vi "GamePanel.vi"() -> ()   [LabVIEW 2025]
uses:
  common/types/network/Move.ctl
  <vilib>/Utility/miscctls.llb/LVPointTypeDef.ctl
  common/types/network/FieldData.ctl
  common/types/network/FoggedFieldCell.ctl
  server/types/TerrainEnum.ctl
  common/types/network/ClientSendData.ctl
  b634419e-299d-4ea9-b051-81e51aeb9912.vi
  d835d933-86fe-443f-b748-a417a8161ed5.vi
  ClientGlobalVariables.vi
panel:
  out "Chain Move":bool=TRUE
  out "MoveSet":set{T1}(c389)
  out "Split":bool=TRUE
  out "CurrentSelectedCell":cluster{"row":i32, "col":i32}
  out "Round Number":dbl
  out "Field Display":picture
  # "Round #"
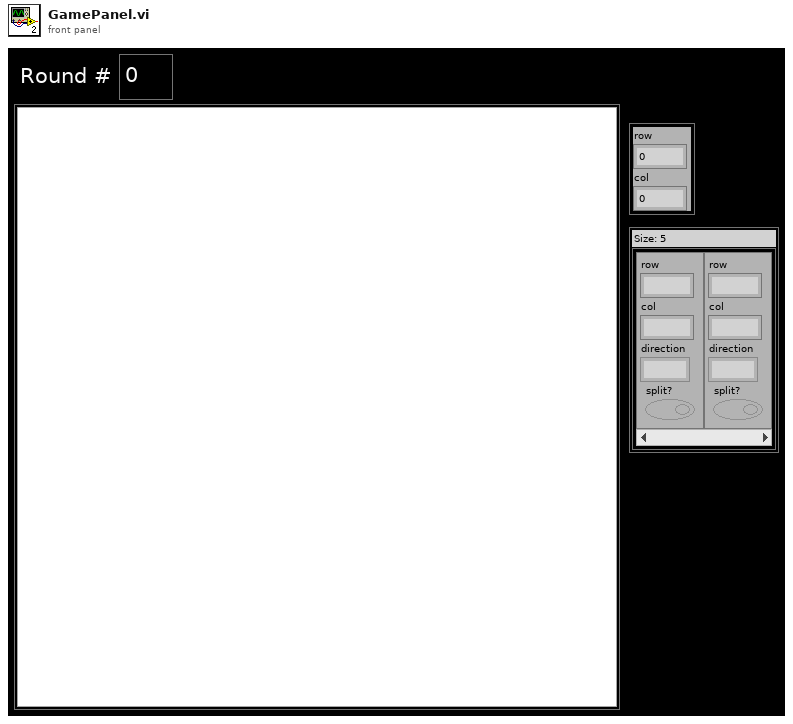
[diagram p1: front panel]
types:
  T1 = typedef "Move.ctl" = cluster{"row":u32, "col":u32, "direction":enum16{"right", "down", "left", "up"}, "split?":bool}
  T2 = typedef "LVPointTypeDef.ctl" = cluster{"Horizontal":i16, "Vertical":i16}
  T3 = typedef "LVPoint32TypeDef.ctl" = cluster{"Horizontal":i32, "Vertical":i32}
  T4 = typedef "LVPositionTypeDef.ctl" = cluster{"Left":i32, "Top":i32}
  T5 = typedef "TerrainEnum.ctl" = enum16{"Plain", "Mountain", "City", "General"}
  T6 = typedef "FoggedFieldCell.ctl" = cluster{"Troops":u32, "Owner":i32, "Terrain":T5, "Fog":bool}
  T7 = typedef "FieldData.ctl" = cluster{"Round":u32, "FoggedFieldArray":T6[][]}
  T8 = typedef "ClientSendData.ctl" = cluster{"Action":string, "Data":string}
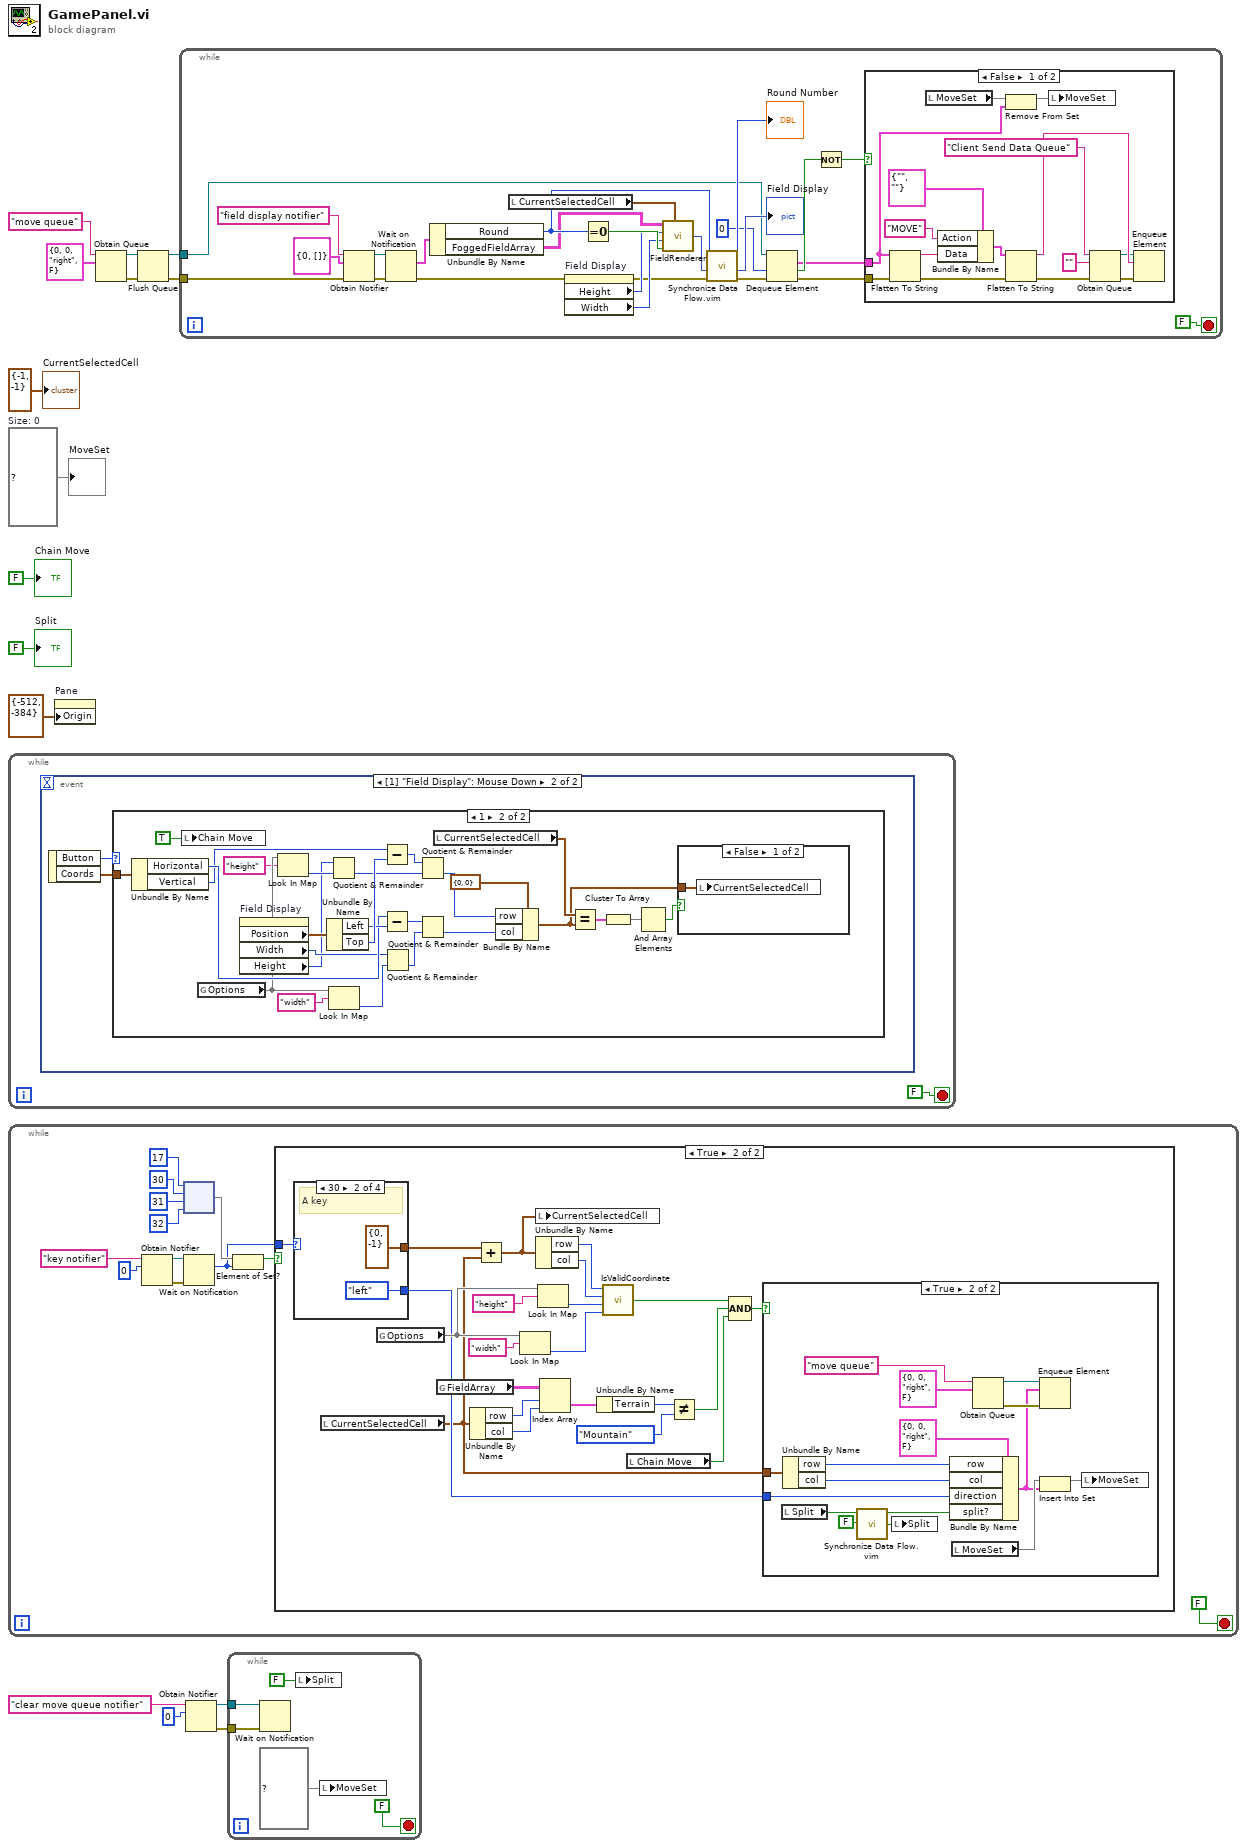
[diagram p0: block diagram]
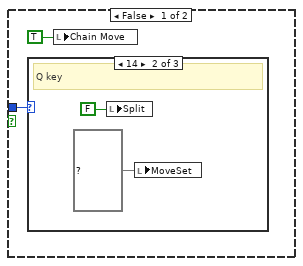
[diagram p2: hidden frame]
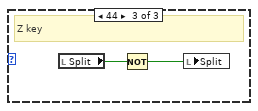
[diagram p4: hidden frame]
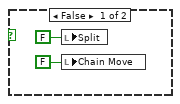
[diagram p5: hidden frame]
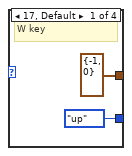
[diagram p6: hidden frame]
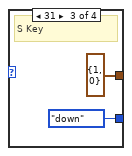
[diagram p7: hidden frame]
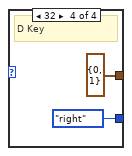
[diagram p8: hidden frame]
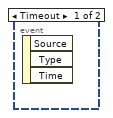
[diagram p9: hidden frame]
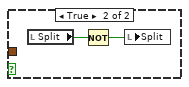
[diagram p11: hidden frame]
diagram:
  w12 = set{T1} {}  # Size: 0
  n1 = while {
    stop <- FALSE stop-if-true
    n2 = event shown="[1] \"Field Display\": Mouse Down" {
      selector: _ -> [_ _]
      dyn-events: _ -> [_ _]
      timeout: _ -> [_ _]
      event Timeout {
        n3 = event-data() -> ()  [unwired: 1 in, 3 out]
      }
      event "Field Display": Mouse Down {
        n4 = event-data() -> ("Button"=w18:u16, "Coords"=w17:T3)  [unwired: 1 in]
        n5 = case shown="1" w18 {
          tunnel: w17 -> [_ w44]
          frame 0, Default {
          }
          frame 1 {
            n6 = Unbundle By Name(w44) -> ("Horizontal"=w35:i32, "Vertical"=w34:i32)
            n7 = local write "Chain Move"(TRUE ("Chain Move")) -> ()
            n8 = global read "ClientGlobalVariables.vi" "Options"() -> (w30:map{string, i32})
            n9 = property on="Field Display" class="Pict"() -> ("Position"=w38:T4, "Width"=w27:u32, "Height"=w24:u32)  [unwired: 2 in, 2 out]
            n10 = Look In Map(map=w30, key="height") -> (value=w25:i32)  [unwired: 1 in, 1 out]
            n11 = Unbundle By Name(w38) -> ("Left"=w36:i32, "Top"=w37:i32)
            n12 = Quotient & Remainder(x=w24, y=w25) -> (floor(x/y)=w23:u32)  [unwired: 1 out]
            n13 = Look In Map(map=w30, key="width") -> (value=w28:i32)  [unwired: 1 in, 1 out]
            n14 = Subtract(x=w34, y=w37) -> (x-y=w32:i32)
            n15 = Subtract(x=w35, y=w36) -> (x-y=w33:i32)
            n16 = Quotient & Remainder(x=w27, y=w28) -> (floor(x/y)=w26:u32)  [unwired: 1 out]
            n17 = Quotient & Remainder(x=w32, y=w23) -> (floor(x/y)=w22:u32)  [unwired: 1 out]
            n18 = Quotient & Remainder(x=w33, y=w26) -> (floor(x/y)=w21:u32)  [unwired: 1 out]
            n19 = local read "CurrentSelectedCell"() -> (w40:cluster{"row":i32, "col":i32})
            n20 = Bundle By Name(cluster=cluster{"row":i32, "col":i32} {"row"=0, "col"=0} ("CurrentSelectedCell"), "row"=w22, "col"=w21) -> (w20:cluster{"row":i32, "col":i32})
            n21 = Equal?(x=w40, y=w20) -> (x = y?=w43:cluster{"row":bool, "col":bool})
            n22 = Cluster To Array(cluster=w43) -> (array=w42:bool[])
            n23 = And Array Elements(Boolean array=w42) -> (logical AND=w41:bool)
            n24 = case shown="False" w41 {
              tunnel: w20 -> [w45 _]
              frame False {
                n25 = local write "CurrentSelectedCell"(w45) -> ()
              }
              frame True {
                n26 = local read "Split"() -> (w47:bool)
                n27 = Not(x=w47) -> (.not. x?=w46:bool)
                n28 = local write "Split"(w46) -> ()
              }
            }
          }
        }
      }
    }
  }
  n29 = while {
    stop <- FALSE stop-if-true
    n30 = Obtain Notifier(name (unnamed)="key notifier", notification data type=i16 0 ("ScanCode")) -> (notifier out=w58:refnum<notifier>, error out=w57:errorcluster)  [unwired: 2 in, 1 out]
    n31 = node(i16 17 ("ScanCode"), i16 30 ("ScanCode"), i16 31 ("ScanCode"), i16 32 ("ScanCode")) -> (w55:set{i16})
    n32 = Wait on Notification(notifier=w58, error in (no error)=w57) -> (notification=w50:i16)  [unwired: 2 in, 3 out]
    n33 = Element of Set?(10:w50, 11:w55) -> (3:w56:bool)
    n34 = case shown="True" w56 {
      tunnel: w50 -> [w61 w87]
      frame False {
        n35 = case shown="14" w61 {
          frame 0, Default {
          }
          frame 14 {
            # "Q key"
            n36 = local write "Split"(FALSE ("Split")) -> ()
            n37 = local write "MoveSet"(set{T1} {} ("MoveSet")) -> ()
          }
          frame 44 {
            # "Z key"
            n38 = local read "Split"() -> (w65:bool)
            n39 = Not(x=w65) -> (.not. x?=w64:bool)
            n40 = local write "Split"(w64) -> ()
          }
        }
        n41 = local write "Chain Move"(TRUE ("Chain Move")) -> ()
      }
      frame True {
        n42 = case shown="30" w87 {
          tunnel: [cluster{"row":i32, "col":i32} {"row"=-1, "col"=0} ("CurrentSelectedCell") cluster{"row":i32, "col":i32} {"row"=0, "col"=-1} ("CurrentSelectedCell") cluster{"row":i32, "col":i32} {"row"=1, "col"=0} ("CurrentSelectedCell") cluster{"row":i32, "col":i32} {"row"=0, "col"=1} ("CurrentSelectedCell")] -> w79
          tunnel: [enum16{"right", "down", "left", "up"}."up" ("direction") enum16{"right", "down", "left", "up"}."left" ("direction") enum16{"right", "down", "left", "up"}."down" ("direction") enum16{"right", "down", "left", "up"}."right" ("direction")] -> w77
          frame 17, Default {
            # "W key"
          }
          frame 30 {
            # "A key"
          }
          frame 31 {
            # "S Key"
          }
          frame 32 {
            # "D Key"
          }
        }
        n43 = local read "CurrentSelectedCell"() -> (w74:cluster{"row":i32, "col":i32})
        n44 = global read "ClientGlobalVariables.vi" "Options"() -> (w84:map{string, i32})
        n45 = global read "ClientGlobalVariables.vi" "FieldArray"() -> (w75:T6[][])
        n46 = Unbundle By Name(w74) -> ("row"=w73:i32, "col"=w72:i32)
        n47 = Add(x=w79, y=w74) -> (x+y=w78:cluster{"row":i32, "col":i32})
        n48 = Look In Map(map=w84, key="width") -> (value=w83:i32)  [unwired: 1 in, 1 out]
        n49 = local write "CurrentSelectedCell"(w78) -> ()
        n50 = Unbundle By Name(w78) -> ("row"=w86:i32, "col"=w85:i32)
        n51 = Look In Map(map=w84, key="height") -> (value=w82:i32)  [unwired: 1 in, 1 out]
        n52 = Index Array(array=w75, index (row)=w73, index (col)=w72) -> (element=w70:T6)
        n53 = Unbundle By Name(w70) -> ("Terrain"=w69:T5)
        n54 = call "IsValidCoordinate.vi"("Width"=w83, "Height"=w82, "Column"=w85, "Row"=w86) -> ("Valid"=w76:bool)
        n55 = local read "Chain Move"() -> (w66:bool)
        n56 = Not Equal?(x=w69, y=TerrainEnum."Mountain") -> (x != y?=w67:bool)
        n57 = Compound Arithmetic op=AND(w76, w67, w66) -> (w71:bool)
        n58 = case shown="True" w71 {
          tunnel: w74 -> [_ w103]
          tunnel: w77 -> [_ w95]
          frame False {
            n59 = local write "Split"(FALSE ("Split")) -> ()
            n60 = local write "Chain Move"(FALSE ("Chain Move")) -> ()
          }
          frame True {
            n61 = local read "Split"() -> (w100:bool)
            n62 = Unbundle By Name(w103) -> ("row"=w102:i32, "col"=w101:i32)
            n63 = call "Synchronize Data Flow.vim"("input 2"=FALSE, "input 1"=w100) -> ("output 2"=w98:bool, "output 1"=w99:bool)  [unwired: 2 in, 2 out]
            n64 = local write "Split"(w98) -> ()
            n65 = Bundle By Name(cluster=T1 {"row"=0, "col"=0, "direction"=enum."right", "split?"=FALSE}, "row"=w102, "col"=w101, "direction"=w95, "split?"=w99) -> (w90:T1)
            n66 = local read "MoveSet"() -> (w105:set{T1})
            n67 = Obtain Queue(name (unnamed)="move queue", element data type=T1 {"row"=0, "col"=0, "direction"=enum."right", "split?"=FALSE}) -> (queue out=w92:refnum<queue>, error out=w91:errorcluster)  [unwired: 3 in, 1 out]
            n68 = Enqueue Element(queue=w92, element=w90, error in (no error)=w91) -> ()  [unwired: 1 in, 3 out]
            n69 = Insert Into Set(10:w90, 11:w105) -> (3:w96:set{T1})  [unwired: 1 out]
            n70 = local write "MoveSet"(w96) -> ()
          }
        }
      }
    }
  }
  n71 = property on="Pane" class="Pane"("Origin"=T2 {"Horizontal"=-512, "Vertical"=-384}) -> ()  [unwired: 2 in, 2 out]
  n72 = Obtain Queue(name (unnamed)="move queue", element data type=T1 {"row"=0, "col"=0, "direction"=enum."right", "split?"=FALSE}) -> (queue out=w5:refnum<queue>, error out=w4:errorcluster)  [unwired: 3 in, 1 out]
  n73 = Flush Queue(queue=w5, error in (no error)=w4) -> (queue out=w3:refnum<queue>, error out=w1:errorcluster)  [unwired: 1 out]
  n74 = while {
    tunnel: w3 -> [w118]
    tunnel: w1 -> [w116]
    stop <- FALSE stop-if-true
    n75 = Obtain Notifier(name (unnamed)="field display notifier", notification data type=T7 {"Round"=0, "FoggedFieldArray"=[]} ("FieldDataCluster"), error in (no error)=w116) -> (notifier out=w136:refnum<notifier>, error out=w135:errorcluster)  [unwired: 1 in, 1 out]
    n76 = Wait on Notification(notifier=w136, error in (no error)=w135) -> (notification=w134:T7, error out=w126:errorcluster)  [unwired: 2 in, 2 out]
    n77 = Unbundle By Name(w134) -> ("Round"=w131:u32, "FoggedFieldArray"=w128:T6[][])
    n78 = local read "CurrentSelectedCell"() -> (w114:cluster{"row":i32, "col":i32})
    n79 = property on="Field Display" class="Pict"(error in=w126) -> (error out=w123:errorcluster, "Height"=w125:u32, "Width"=w124:u32)  [unwired: 1 in, 1 out]
    n80 = Equal To 0?(x=w131) -> (x = 0?=w129:bool)
    n81 = call "FieldRenderer.vi"("CurrentSelectedCell"=w114, "FirstCall?"=w129, "FieldWidth"=w124, "FieldHeight"=w125, "FieldArray"=w128) -> ("FieldDisplay"=w130:picture)  [unwired: 1 in]
    n82 = call "Synchronize Data Flow.vim"("input 4"=w123, "input 3"=w130, "input 2"=w131) -> ("output 4"=w117:errorcluster, "output 3"=→"Field Display":picture, "output 2"=→"Round Number":u32)  [unwired: 1 in, 1 out]
    n83 = Dequeue Element(queue=w118, timeout in ms (-1)=0, error in (no error)=w117) -> (element=w119:T1, timed out?=w120:bool, error out=w121:errorcluster)  [unwired: 1 out]
    n84 = Not(x=w120) -> (.not. x?=w115:bool)
    n85 = case shown="False" w115 {
      tunnel: w119 -> [w140 _]
      tunnel: w121 -> [w153 _]
      frame False {
        n86 = Flatten To String(anything=w140, error in (no error)=w153) -> (data string=w150:string, error out=w148:errorcluster)  [unwired: 2 in, 1 out]
        n87 = local read "MoveSet"() -> (w141:set{T1})
        n88 = Bundle By Name(cluster=T8 {"Action"="", "Data"=""} ("ClientSendData"), "Action"="MOVE", "Data"=w150) -> (w149:T8)
        n89 = Remove From Set(10:w140, 11:w141) -> (3:w139:set{T1})  [unwired: 1 out]
        n90 = Flatten To String(anything=w149, error in (no error)=w148) -> (data string=w144:string, error out=w145:errorcluster)  [unwired: 2 in, 1 out]
        n91 = local write "MoveSet"(w139) -> ()
        n92 = Obtain Queue(name (unnamed)="Client Send Data Queue", element data type="", error in (no error)=w145) -> (queue out=w143:refnum<queue>, error out=w142:errorcluster)  [unwired: 2 in, 1 out]
        n93 = Enqueue Element(queue=w143, element=w144, error in (no error)=w142) -> ()  [unwired: 1 in, 3 out]
      }
      frame True {
      }
    }
  }
  n94 = Obtain Notifier(name (unnamed)="clear move queue notifier", notification data type=0) -> (notifier out=w8:refnum<notifier>, error out=w7:errorcluster)  [unwired: 2 in, 1 out]
  n95 = while {
    tunnel: w8 -> [w156]
    tunnel: w7 -> [w155]
    stop <- FALSE stop-if-true
    n96 = Wait on Notification(notifier=w156, error in (no error)=w155) -> ()  [unwired: 2 in, 4 out]
    n97 = local write "Split"(FALSE ("Split")) -> ()
    n98 = local write "MoveSet"(set{T1} {} ("MoveSet")) -> ()
  }
  "CurrentSelectedCell" <- cluster{"row":i32, "col":i32} {"row"=-1, "col"=-1} ("CurrentSelectedCell")
  "Split" <- FALSE ("Split")
  "MoveSet" <- w12
  "Chain Move" <- FALSE ("Split")
